vi "Open Gearbox.vi"(0 "Digital Module (Module 1)":T3, 1 "Invert Motor 1":bool, 2 "Invert Motor 2":bool, 3 "Invert Motor 3":bool, 5 "Motor 1":T4, 7 "Motor 2":T4=enum."PWM 2", 9 "Motor 3":T4=enum."PWM 3", 11 "error in":errorcluster) -> (4 "Gearbox data":T1, 15 "error out":errorcluster)   [LabVIEW 2013]
uses:
  <vilib>/Rock Robotics/SystemInterfaces/DIO/FPGA_DIOPWMChannel.ctl
  <vilib>/Rock Robotics/SystemInterfaces/Typedef/FPGA_TypedefDigitalModule.ctl
  GearBox Typedef.ctl
  <vilib>/Rock Robotics/WPI/MotorControl/WPI_MotorControlDeviceRef.ctl
  <vilib>/Rock Robotics/WPI/PWM/WPI_PWMDeadband.ctl
  <vilib>/Rock Robotics/WPI/CAN/Jaguar/SubVIs/WPI_CANJaguar_ControlMode.ctl
  <vilib>/Rock Robotics/WPI/PWM/WPI_PWMTransform_ConPane.ctl
  <vilib>/Rock Robotics/WPI/MotorControl/WPI_MotorControlOpen Talon.vi
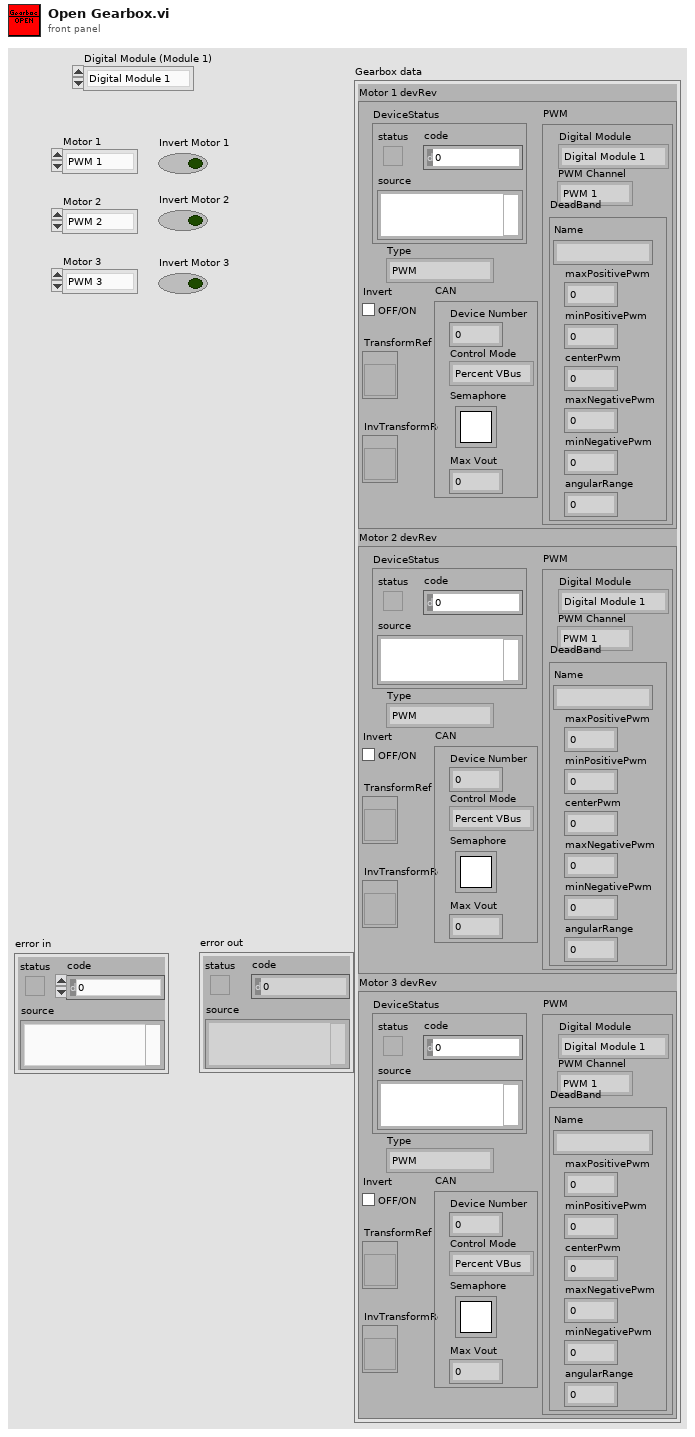
[diagram p1: front panel]
types:
  T1 = typedef "GearBox Typedef.ctl" = cluster{"Motor 1 devRev":T2, "Motor 2 devRev":T2, "Motor 3 devRev":T2}
  T2 = typedef "WPI_MotorControlDeviceRef.ctl" = cluster{"DeviceStatus":errorcluster, "Type":enum16{"PWM", "CAN"}, "PWM":cluster{"Digital Module":T3, "PWM Channel":T4, "DeadBand":T5}, "CAN":cluster{"Device Number":u8, "Control Mode":T6, "Semaphore":T7, "Max Vout":dbl}, "Invert":bool, "TransformRef":T8, "InvTransformRef":T8}
  T3 = typedef "FPGA_TypedefDigitalModule.ctl" = enum16{"Digital Module 1", "Digital Module 2"}
  T4 = typedef "FPGA_DIOPWMChannel.ctl" = enum8{"PWM 1", "PWM 2", "PWM 3", "PWM 4", "PWM 5", "PWM 6", "PWM 7", "PWM 8", "PWM 9", "PWM 10", "Invalid"}
  T5 = typedef "WPI_PWMDeadband.ctl" = cluster{"Name":string, "maxPositivePwm":i32, "minPositivePwm":i32, "centerPwm":i32, "maxNegativePwm":i32, "minNegativePwm":i32, "angularRange":u16}
  T6 = typedef "WPI_CANJaguar_ControlMode.ctl" = enum8{"Percent VBus", "Current", "Speed", "Position", "Voltage"}
  T7 = typedef "Semaphore RefNum" = refnum<k1>
  T8 = typedef "WPI_PWMTransform_ConPane.ctl" = refnum<vi>
  T9 = cluster{"MotorControlDeviceRef":T2, "MotorControlDeviceRef":T2, "MotorControlDeviceRef":T2}
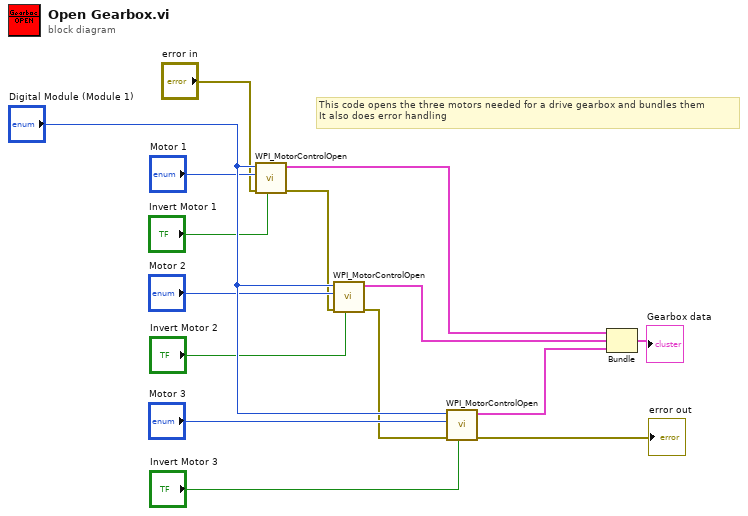
[diagram p0: block diagram]
diagram:
  # "This code opens the three motors needed for a drive gearbox and bundles them\nIt also does error handling"
  n1 = call-poly <vilib>:"WPI_MotorControlOpen.vi"("Invert"="Invert Motor 1", "error in (no error)"="error in", "PWM Channel"="Motor 1", "Digital Module (Module 1)"="Digital Module (Module 1)") -> ("error out"=w5:errorcluster, "MotorControlDeviceRef"=w8:T2)  [unwired: 6 in]
  n2 = call-poly <vilib>:"WPI_MotorControlOpen.vi"("Invert"="Invert Motor 2", "error in (no error)"=w5, "PWM Channel"="Motor 2", "Digital Module (Module 1)"="Digital Module (Module 1)") -> ("error out"=w4:errorcluster, "MotorControlDeviceRef"=w7:T2)  [unwired: 6 in]
  n3 = call-poly <vilib>:"WPI_MotorControlOpen.vi"("Invert"="Invert Motor 3", "error in (no error)"=w4, "PWM Channel"="Motor 3", "Digital Module (Module 1)"="Digital Module (Module 1)") -> ("error out"=→"error out":errorcluster, "MotorControlDeviceRef"=w6:T2)  [unwired: 6 in]
  n4 = Bundle("MotorControlDeviceRef"=w8, "MotorControlDeviceRef"=w7, "MotorControlDeviceRef"=w6) -> (→"Gearbox data":T9)  [unwired: 1 in]
